vi "nrm2 - Vector 2-Norm.vi"   [LabVIEW 2020, in "NI_AALBLAS.lvlib"]
doc: "Calculates the Euclidean norm of a vector."
uses:
  NI_AALBLAS.lvlib
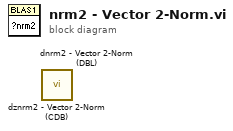
[diagram p0: block diagram]
diagram:
  n1 = call "dznrm2 - Vector 2-Norm (CDB).vi"() -> ()  [unwired: 10 in, 2 out]
  n2 = call "dnrm2 - Vector 2-Norm (DBL).vi"() -> ()  [unwired: 10 in, 2 out]
